vi "Remove aspas.vi"(11 "textoComAspas":string) -> (3 "textoEntreAspas":string)   [LabVIEW 2012]
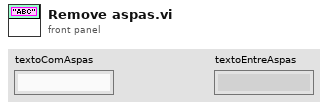
[diagram p1: front panel]
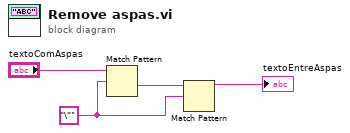
[diagram p0: block diagram]
diagram:
  w2 = "\"" ("regular expression")
  n1 = Match Pattern(string="textoComAspas", regular expression=w2) -> (after substring=w3:string)  [unwired: 1 in, 3 out]
  n2 = Match Pattern(string=w3, regular expression=w2) -> (before substring=→"textoEntreAspas":string)  [unwired: 1 in, 3 out]
